vi "QE Reset 1 Chan.vi"(8 "Error In":errorcluster, 10 "QE Channel":u8, 11 "LINX Resource":T1) -> (0 "Error Out":errorcluster, 3 "LINX Resource":T1)   [LabVIEW 2013, in "LVH-LINX.lvlib"]
doc: "Set counter value to 0 for the specified quadrature encoder channel."
uses:
  LVH-LINX.lvlib
  Private/Type Defs/LINX Ref.ctl
  Private/Type Defs/Platform.ctl
  Private/Type Defs/Interface.ctl
  Private/Device/Type Defs/LINX Device Config.ctl
  Private/Device/Type Defs/TCP Config.ctl
  Private/Device/Type Defs/Channels.ctl
  Private/Device/Device.lvlib
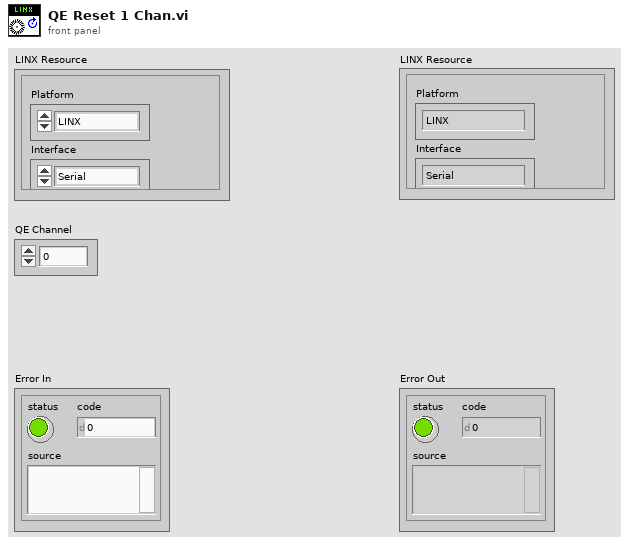
[diagram p1: front panel]
types:
  T1 = typedef "LVH-LINX.lvlib/LINX Ref.ctl" = cluster{"Platform":T2, "Interface":T3, "LINX Device Config":T4}
  T2 = typedef "LVH-LINX.lvlib/Platform.ctl" = enum16{"LINX", "myRIO"}
  T3 = typedef "LVH-LINX.lvlib/Interface.ctl" = enum16{"Serial", "TCP"}
  T4 = typedef "LVH-LINX.lvlib/Device.lvlib/LINX Device Config.ctl" = cluster{"Interface":T3, "COM Port":refnum<visa-resource-name>, "TCP Configuration":T5, "Device Family":u8, "Device ID":u8, "Device Name":string, "TCP Ref":refnum<k5>, "Channels":T6}
  T5 = typedef "LVH-LINX.lvlib/Device.lvlib/TCP Config.ctl" = cluster{"IP Address":string, "Port":u16}
  T6 = typedef "LVH-LINX.lvlib/Channels.ctl" = cluster{"DI Channels":u8[], "DO Channels":u8[], "AI":u8[], "AO":u8[], "PWM":u8[], "QE":u8[], "UART":u8[], "I2C 2":u8[], "SPI":u8[], "CAN":u8[], "AI Ref (V)":dbl, "AO Resolution (Bits)":u8, "AO Ref (V)":dbl}
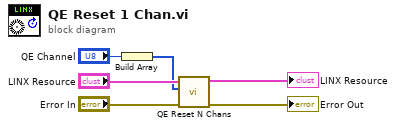
[diagram p0: block diagram]
diagram:
  n1 = Build Array("QE Channel") -> (w3:u8[])
  n2 = call "QE Reset N Chans.vi"("Error In"="Error In", "QE Channels"=w3, "LINX Resource"="LINX Resource") -> ("Error Out"=→"Error Out":errorcluster, "LINX Resource"=→"LINX Resource":T1)  [unwired: 7 in]
